vi "Autonomous Independent.vi"   [LabVIEW 2017]
doc: "This VI is called when autonomous begins, and will automatically be terminated when autonomous ends. You can carry out timed or sensor driven robot movement independently without needing to return to the caller."
uses:
  <vilib>/Rock Robotics/WPI/Utilities/WPI_GetSetVariantRefNum.vi
  <vilib>/Rock Robotics/Network Tables/NT Read Boolean.vi
  <vilib>/Rock Robotics/Network Tables/NT Read Number.vi
  <vilib>/Rock Robotics/Network Tables/NT Write String.vi
types:
  T1 = typedef "WPI_CompressorDevRef.ctl" = cluster{"DevStatus":errorcluster, "Pneumatics Control Module":u8}
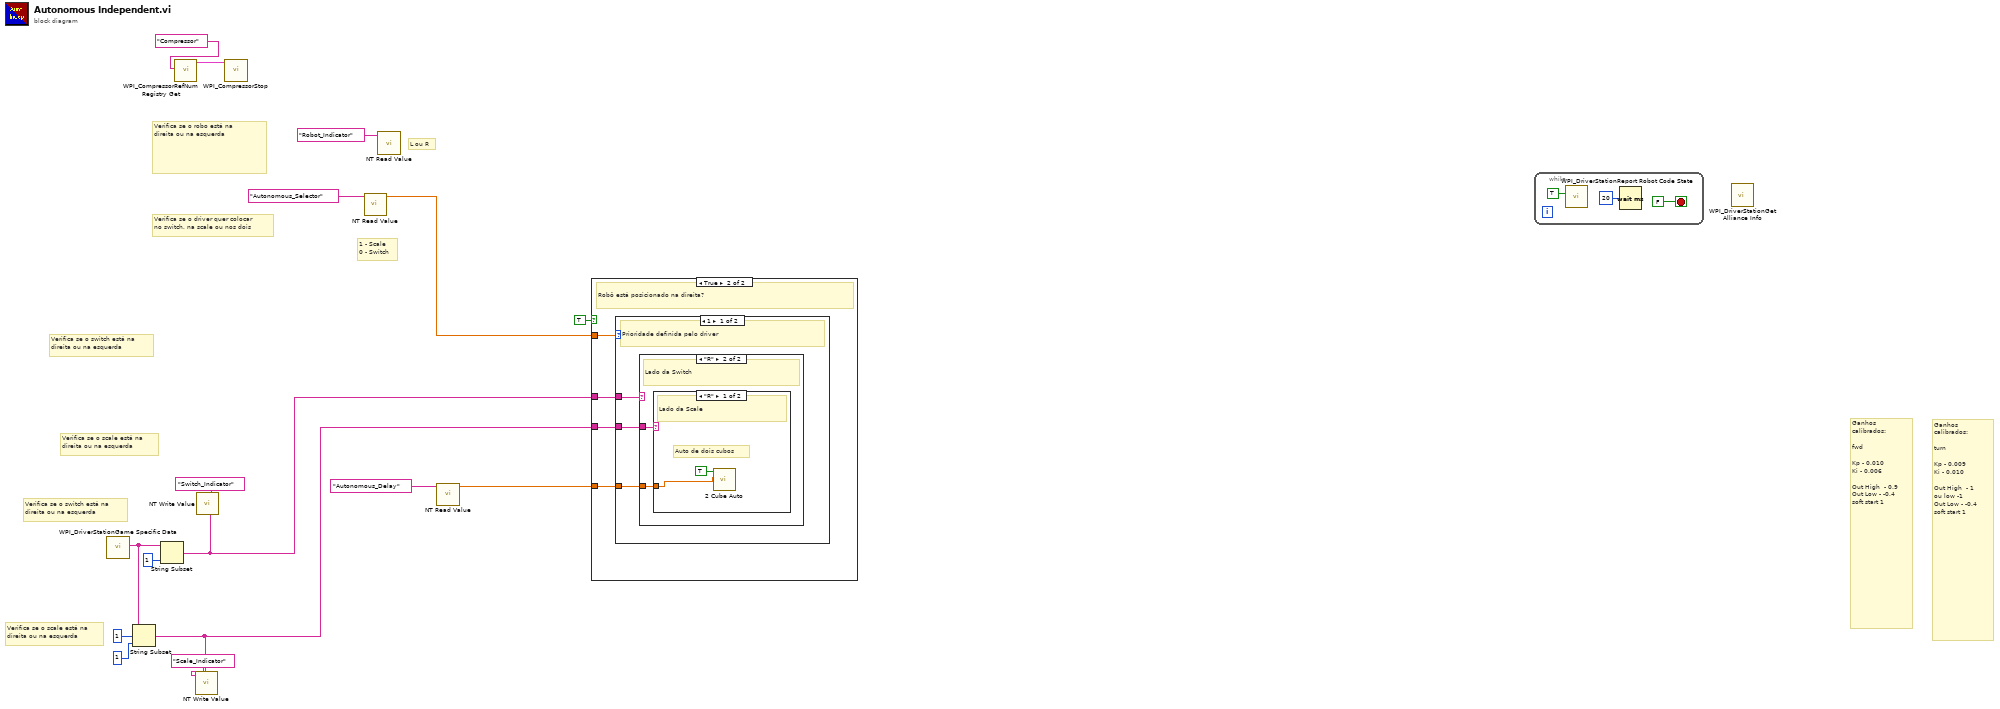
[diagram p0: block diagram]
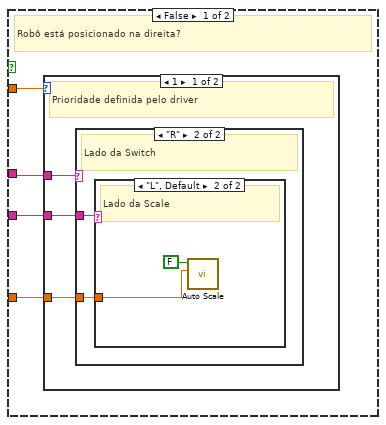
[diagram p2: hidden frame]
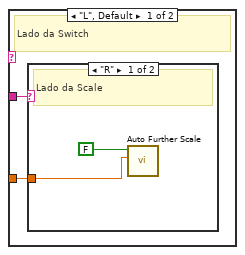
[diagram p3: hidden frame]
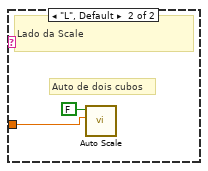
[diagram p4: hidden frame]
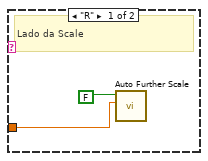
[diagram p5: hidden frame]
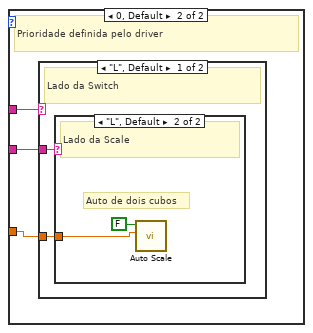
[diagram p6: hidden frame]
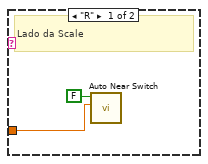
[diagram p7: hidden frame]
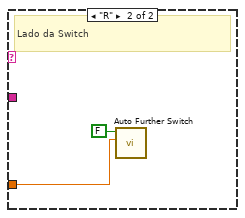
[diagram p8: hidden frame]
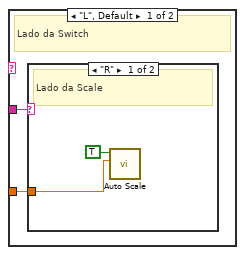
[diagram p9: hidden frame]
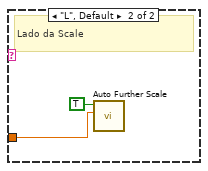
[diagram p10: hidden frame]
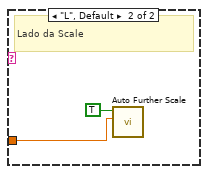
[diagram p11: hidden frame]
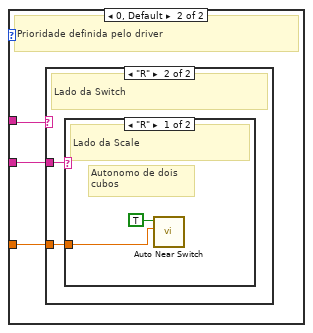
[diagram p12: hidden frame]
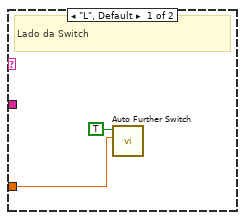
[diagram p13: hidden frame]
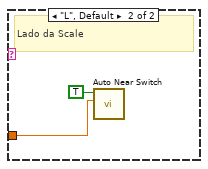
[diagram p14: hidden frame]
diagram:
  # "Verifica se o scale está na\ndireita ou na esquerda"
  # "Verifica se o switch está na\ndireita ou na esquerda"
  # "1 - Scale\n0 - Switch"
  # "L ou R"
  # "Verifica se o driver quer colocar\nno switch, na scale ou nos dois"
  # "Verifica se o scale está na\ndireita ou na esquerda"
  # "Verifica se o switch está na\ndireita ou na esquerda"
  # "Verifica se o robo está na\ndireita ou na esquerda"
  # "Ganhos calibrados:\n\nturn\n\nKp - 0.009\nKi - 0.010\n\nOut High  - 1\nou low -1\nOut Low - -0.4\nsoft start 1"
  # "Ganhos calibrados:\n\nfwd\n\nKp - 0.010\nKi - 0.006\n\nOut High  - 0.9\nOut Low - -0.4\nsoft start 1"
  n1 = call <vilib>:"WPI_DriverStationGame Specific Data.vi"() -> ("Game Specific Data"=w9:string)  [unwired: 11 in]
  n2 = String Subset(string=w9, offset (0)=1, length (rest)=1 ("length (rest)")) -> (substring=w1:string)
  n3 = String Subset(string=w9, length (rest)=1 ("length (rest)")) -> (substring=w2:string)  [unwired: 1 in]
  n4 = call <vilib>:"WPI_CompressorRefNum Registry Get.vi"("refnum name"="Compressor") -> ("CompressorDevRef"=w16:T1)  [unwired: 9 in, 1 out]
  n5 = call-poly <vilib>:"NT Write Value.vi"("String"=w1, "Name"="Scale_Indicator") -> ()  [unwired: 9 in, 1 out]
  n6 = call-poly <vilib>:"NT Write Value.vi"("String"=w2, "Name"="Switch_Indicator") -> ()  [unwired: 9 in, 1 out]
  n7 = call <vilib>:"WPI_CompressorStop.vi"("CompressorDevRef"=w16) -> ()  [unwired: 9 in, 2 out]
  n8 = call-poly <vilib>:"NT Read Value.vi"("Name"="Autonomous_Selector") -> ("Numeric"=w14:dbl)  [unwired: 9 in, 1 out]
  n9 = call-poly <vilib>:"NT Read Value.vi"("Name"="Robot_Indicator") -> ()  [unwired: 9 in, 2 out]
  n10 = call-poly <vilib>:"NT Read Value.vi"("Name"="Autonomous_Delay") -> ("Numeric"=w10:dbl)  [unwired: 9 in, 1 out]
  n11 = case shown="True" TRUE {
    tunnel: w14 -> [w20 w50]
    tunnel: w2 -> [w19 w49]
    tunnel: w1 -> [w18 w48]
    tunnel: w10 -> [w17 w47]
    frame False {
      # "Robô está posicionado na direita?"
      n12 = case shown="1" w20 {
        tunnel: w19 -> [w23 w38]
        tunnel: w18 -> [w22 w37]
        tunnel: w17 -> [w21 w36]
        frame 1 {
          # "Prioridade definida pelo driver"
          n13 = case shown="\"R\"" w23 {
            tunnel: w22 -> [w25 w31]
            tunnel: w21 -> [w24 w30]
            frame "L", Default {
              # "Lado da Switch"
              n14 = case shown="\"R\"" w25 {
                tunnel: w24 -> [w26 w28]
                frame "R" {
                  # "Lado da Scale"
                  n15 = call "Auto Further Scale.vi"("Time to wait (min 50ms)"=w26, "Right?"=FALSE) -> ()  [unwired: 10 in]
                }
                frame "L", Default {
                  # "Auto de dois cubos"
                  # "Lado da Scale"
                  n16 = call "Auto Scale.vi"("Time to wait (min 50ms)"=w28, "Right?"=FALSE) -> ()  [unwired: 10 in]
                }
              }
            }
            frame "R" {
              # "Lado da Switch"
              n17 = case shown="\"L\", Default" w31 {
                tunnel: w30 -> [w32 w34]
                frame "R" {
                  # "Lado da Scale"
                  n18 = call "Auto Further Scale.vi"("Time to wait (min 50ms)"=w32, "Right?"=FALSE) -> ()  [unwired: 10 in]
                }
                frame "L", Default {
                  # "Lado da Scale"
                  n19 = call "Auto Scale.vi"("Time to wait (min 50ms)"=w34, "Right?"=FALSE) -> ()  [unwired: 10 in]
                }
              }
            }
          }
        }
        frame 0, Default {
          # "Prioridade definida pelo driver"
          n20 = case shown="\"L\", Default" w38 {
            tunnel: w37 -> [w40 _]
            tunnel: w36 -> [w39 w45]
            frame "L", Default {
              # "Lado da Switch"
              n21 = case shown="\"L\", Default" w40 {
                tunnel: w39 -> [w41 w43]
                frame "R" {
                  # "Lado da Scale"
                  n22 = call "Auto Near Switch.vi"("Time to wait (min 50ms)"=w41, "Right?"=FALSE) -> ()  [unwired: 9 in]
                }
                frame "L", Default {
                  # "Auto de dois cubos"
                  # "Lado da Scale"
                  n23 = call "Auto Scale.vi"("Time to wait (min 50ms)"=w43, "Right?"=FALSE) -> ()  [unwired: 10 in]
                }
              }
            }
            frame "R" {
              # "Lado da Switch"
              n24 = call "Auto Further Switch.vi"("Time to wait (min 50ms)"=w45, "Right?"=FALSE) -> ()  [unwired: 10 in]
            }
          }
        }
      }
    }
    frame True {
      # "Robô está posicionado na direita?"
      n25 = case shown="1" w50 {
        tunnel: w49 -> [w53 w68]
        tunnel: w48 -> [w52 w67]
        tunnel: w47 -> [w51 w66]
        frame 1 {
          # "Prioridade definida pelo driver"
          n26 = case shown="\"R\"" w53 {
            tunnel: w52 -> [w55 w61]
            tunnel: w51 -> [w54 w60]
            frame "L", Default {
              # "Lado da Switch"
              n27 = case shown="\"R\"" w55 {
                tunnel: w54 -> [w56 w58]
                frame "R" {
                  # "Lado da Scale"
                  n28 = call "Auto Scale.vi"("Time to wait (min 50ms)"=w56, "Right?"=TRUE) -> ()  [unwired: 10 in]
                }
                frame "L", Default {
                  # "Lado da Scale"
                  n29 = call "Auto Further Scale.vi"("Time to wait (min 50ms)"=w58, "Right?"=TRUE) -> ()  [unwired: 10 in]
                }
              }
            }
            frame "R" {
              # "Lado da Switch"
              n30 = case shown="\"R\"" w61 {
                tunnel: w60 -> [w62 w64]
                frame "R" {
                  # "Auto de dois cubos"
                  # "Lado da Scale"
                  n31 = call "2 Cube Auto.vi"("Time to wait (min 50ms)"=w62, "Right?"=TRUE) -> ()  [unwired: 10 in]
                }
                frame "L", Default {
                  # "Lado da Scale"
                  n32 = call "Auto Further Scale.vi"("Time to wait (min 50ms)"=w64, "Right?"=TRUE) -> ()  [unwired: 10 in]
                }
              }
            }
          }
        }
        frame 0, Default {
          # "Prioridade definida pelo driver"
          n33 = case shown="\"R\"" w68 {
            tunnel: w67 -> [_ w72]
            tunnel: w66 -> [w69 w71]
            frame "L", Default {
              # "Lado da Switch"
              n34 = call "Auto Further Switch.vi"("Time to wait (min 50ms)"=w69, "Right?"=TRUE) -> ()  [unwired: 10 in]
            }
            frame "R" {
              # "Lado da Switch"
              n35 = case shown="\"R\"" w72 {
                tunnel: w71 -> [w73 w75]
                frame "R" {
                  # "Autonomo de dois \ncubos"
                  # "Lado da Scale"
                  n36 = call "Auto Near Switch.vi"("Time to wait (min 50ms)"=w73, "Right?"=TRUE) -> ()  [unwired: 9 in]
                }
                frame "L", Default {
                  # "Lado da Scale"
                  n37 = call "Auto Near Switch.vi"("Time to wait (min 50ms)"=w75, "Right?"=TRUE) -> ()  [unwired: 9 in]
                }
              }
            }
          }
        }
      }
    }
  }
  n38 = while {
    stop <- FALSE stop-if-true
    n39 = call <vilib>:"WPI_DriverStationReport Robot Code State.vi"("Autonomous"=TRUE) -> ()  [unwired: 10 in, 1 out]
    n40 = Wait (ms)(milliseconds to wait=u32 20) -> ()  [unwired: 1 out]
  }
  n41 = call <vilib>:"WPI_DriverStationGet Alliance Info.vi"() -> ()  [unwired: 12 out]
